vi "ForceSerial.vi"(0 "reference in":refnum<class "DUT_Handler_Base.lvclass">, 5 "SN":string, 7 "BN":string, 9 "ID":u32, 11 "error in (no error)":errorcluster) -> (4 "reference in":refnum<class "DUT_Handler_Base.lvclass">, 15 "error out":errorcluster)   [LabVIEW 2017]
uses:
  DUT_Handler_Base.lvclass
  Action.ctl
  EventData.ctl
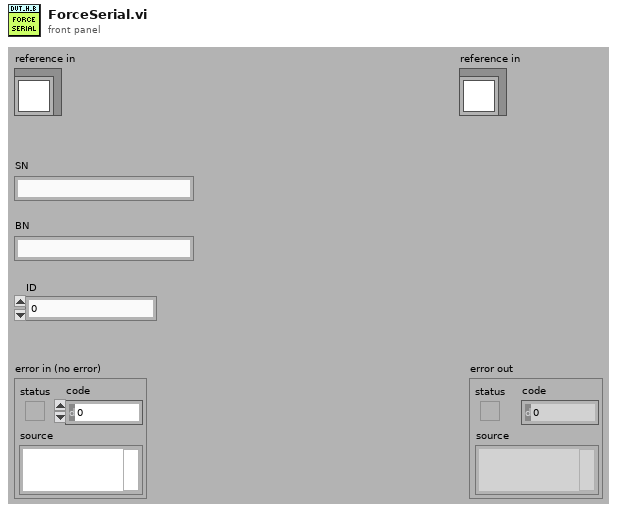
[diagram p1: front panel]
types:
  T1 = typedef "DUT_Handler_Bailey.lvlib/DUT_Handler_Base.lvclass/EventData.ctl" = cluster{"Action":T2, "SN":string, "BN":string, "DUT__ID":u32}
  T2 = typedef "DUT_Handler_Bailey.lvlib/DUT_Handler_Base.lvclass/Action.ctl" = enum16{"Start", "Abort", "Finish", "Fault"}
  T3 = typedef "DUT_Handler_Bailey.lvlib/DUT_Handler_Base.lvclass/ObjectAttributes.ctl" = cluster{"Config":T4, "Event":refnum<user-event>}
  T4 = typedef "DUT_Handler_Bailey.lvlib/DUT_Handler_Base.lvclass/Config.ctl" = cluster{"default":string}
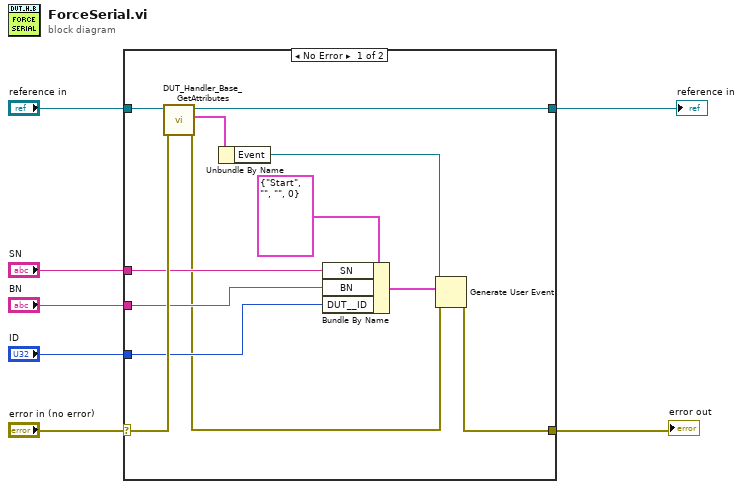
[diagram p0: block diagram]
diagram:
  n1 = case shown="No Error" "error in (no error)" {
    selector: "error in (no error)" -> [w19 w21]
    tunnel: [w9 w21] -> w6
    tunnel: [w16 w20] -> w4
    tunnel: "reference in" -> [w17 w20]
    tunnel: "SN" -> [w13 _]
    tunnel: "BN" -> [w12 _]
    tunnel: "ID" -> [w11 _]
    frame No Error {
      n2 = call "DUT_Handler_Base_GetAttributes.vi"("error in (no error)"=w19, "reference in"=w17) -> ("error out"=w10:errorcluster, "Data"=w18:T3, "reference out"=w16:refnum<class "DUT_Handler_Base.lvclass">)  [unwired: 6 in, 1 out]
      n3 = Unbundle By Name(w18) -> ("Event"=w15:refnum<user-event>)
      n4 = Bundle By Name(cluster=T1 {"Action"=enum."Start", "SN"="", "BN"="", "DUT__ID"=0} ("event data"), "SN"=w13, "BN"=w12, "DUT__ID"=w11) -> (w8:T1)
      n5 = Generate User Event(user event=w15, event data cluster=w8, error in=w10) -> (error out=w9:errorcluster)  [unwired: 1 in, 1 out]
    }
    frame Error {
    }
  }
  "error out" <- w6
  "reference in" <- w4
